vi "addCmd.vi"(8 "error in (no error)":errorcluster, 10 "Command":refnum<class "Command.lvclass">, 11 "Subsystem in":refnum<class "Subsystem.lvclass">) -> (0 "error out":errorcluster, 3 "Subsystem out":refnum<class "Subsystem.lvclass">)   [LabVIEW 2017, in "Subsystem.lvclass"]
uses:
  <userlib>/836-Library/Robot/Subsystem/Subsystem.lvclass
  <userlib>/836-Library/Robot/Command/Command.lvclass
  <userlib>/836-Library/Robot/Subsystem/Subsystem.lvclass/Subsystem.ctl
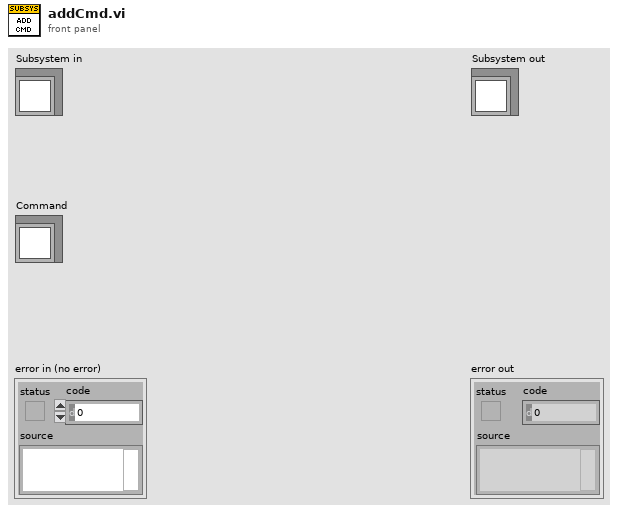
[diagram p1: front panel]
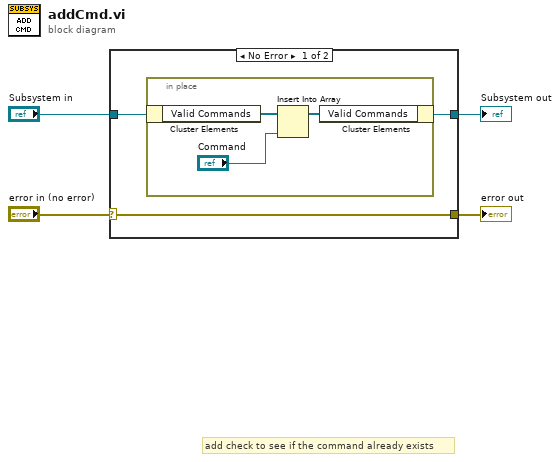
[diagram p0: block diagram]
diagram:
  # "add check to see if the command already exists"
  n1 = case shown="No Error" "error in (no error)" {
    selector: "error in (no error)" -> [w5 w12]
    tunnel: [w5 w12] -> w3
    tunnel: [w6 w11] -> w2
    tunnel: "Subsystem in" -> [w7 w11]
    frame No Error {
      n2 = in-place {
        n3 = in-place-cluster #1(w7) -> ("Valid Commands"=w10:refnum<class "Command.lvclass">[])
        n4 = Insert Into Array(array=w10, new element="Command") -> (w9:refnum<class "Command.lvclass">[])  [unwired: 1 in]
        n5 = in-place-cluster #1("Valid Commands"=w9) -> (w6:refnum<class "Subsystem.lvclass">)
      }
    }
    frame Error {
    }
  }
  "error out" <- w3
  "Subsystem out" <- w2
